vi "Tag.seek_lua.vi"(5 "LuaVIEW reference":T1) -> (15 "error out":errorcluster)   [LabVIEW 2012]
doc: "Seek the read_index relative to its current value. This changes the read position in the tag buffer that will be used during the next <code>read</code>. A positive delta moves the read position to later points, a negative delta moves the read position to earlier points. Note that the number of available earlier points equals the minimum of either the tag's buffer capacity or the number of written points. Therefore do not move the read_index backward too far or else the subsequent <code>read</code> will fail.\nParameters:\nobj:tag\nI32:delta, number of point positions by which to change the read_index.\nErrors:\nDead or invalid tag object."
uses:
  luaview/typedefs/t_LuaVIEW Reference.ctl
  luaview/subvis/private/LuaVIEW Pull (object).vi
  luaview/subvis/private/LuaVIEW Pull (I32).vi
  luaview/subvis/private/LuaVIEW Push (I32).vi
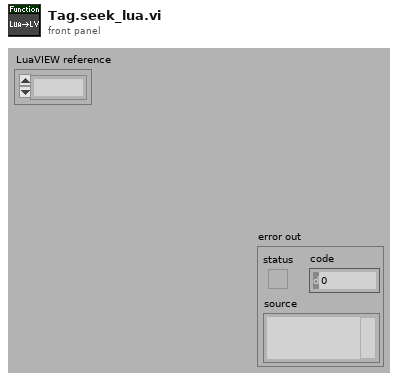
[diagram p1: front panel]
types:
  T1 = typedef "t_LuaVIEW Reference.ctl" = refnum<k1>
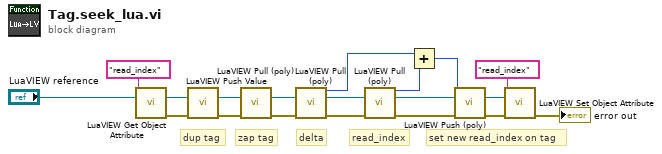
[diagram p0: block diagram]
diagram:
  # "delta"
  # "set new read_index on tag"
  # "dup tag"
  # "zap tag"
  # "read_index"
  n1 = call "LuaVIEW Get Object Attribute.vi"("key"="read_index", "LuaVIEW reference in"="LuaVIEW reference") -> ("LuaVIEW reference out"=w15:T1, "error out"=w16:errorcluster)  [unwired: 12 in]
  n2 = call "LuaVIEW Push Value.vi"("LuaVIEW reference in"=w15, "error in (no error)"=w16) -> ("LuaVIEW reference out"=w14:T1, "error out"=w13:errorcluster)  [unwired: 12 in]
  n3 = call-poly "LuaVIEW Pull (poly).vi"("LuaVIEW reference in"=w14, "error in (no error)"=w13) -> ("LuaVIEW reference out"=w17:T1, "error out"=w19:errorcluster)  [unwired: 10 in, 2 out]
  n4 = call-poly "LuaVIEW Pull (poly).vi"("LuaVIEW reference in"=w17, "error in (no error)"=w19) -> ("I32"=w4:i32, "LuaVIEW reference out"=w8:T1, "error out"=w9:errorcluster)  [unwired: 11 in]
  n5 = call-poly "LuaVIEW Pull (poly).vi"("LuaVIEW reference in"=w8, "error in (no error)"=w9) -> ("I32"=w5:i32, "LuaVIEW reference out"=w7:T1, "error out"=w6:errorcluster)  [unwired: 11 in]
  n6 = Add(x=w4, y=w5) -> (x+y=w3:i32)
  n7 = call-poly "LuaVIEW Push (poly).vi"("I32"=w3, "LuaVIEW reference in"=w7, "error in (no error)"=w6) -> ("LuaVIEW reference out"=w11:T1, "error out"=w12:errorcluster)  [unwired: 11 in]
  n8 = call "LuaVIEW Set Object Attribute.vi"("key"="read_index", "LuaVIEW reference in"=w11, "error in (no error)"=w12) -> ("error out"=→"error out":errorcluster)  [unwired: 11 in, 1 out]
